vi "Get RT by Name.vi"(8 "error in":errorcluster, 10 "name":string, 11 "1553channel ref in":refnum<k24>) -> (0 "error out":errorcluster, 1 "remote terminal":refnum<k24>, 2 "found":bool, 3 "1553channel ref out":refnum<k24>)   [LabVIEW 2020, in "Ballard_1553_Hardware_ni.lvlib"]
uses:
  Ballard_1553_Hardware_ni.lvlib
  C:/Users/Administrator/Desktop/GIT/Ballard-MIL-STD-1553-Custom-Device/Source/System Explorer/SubVIs/Parse XML Ballard/1.2/BTIXML_SerDes.dll
  Ballard-MIL-STD-1553-Custom-Device/Source/System Explorer/SubVIs/Parse XML Ballard/1.2/BTIXML_SerDes.dll
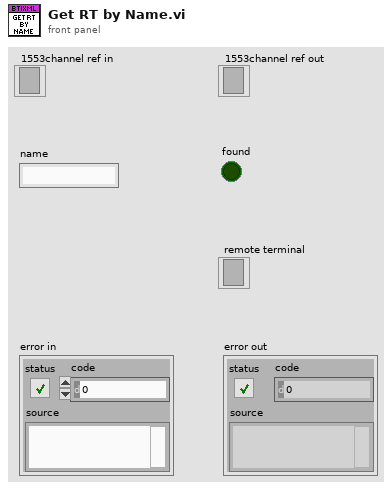
[diagram p1: front panel]
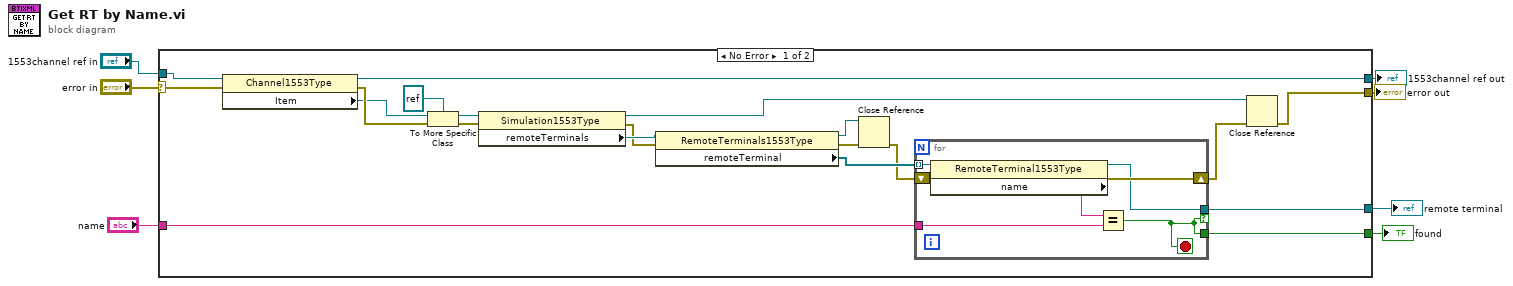
[diagram p0: block diagram]
diagram:
  n1 = case shown="No Error" "error in" {
    selector: "error in" -> [w18 w35]
    tunnel: [w19 w35] -> w7
    tunnel: [w27 w36] -> w6
    tunnel: "1553channel ref in" -> [w26 w36]
    tunnel: "name" -> [w11 _]
    tunnel: [w10 _] -> w2
    tunnel: [w8 _] -> w1
    frame No Error {
      n2 = property class="Channel1553Type"(reference=w26, error in=w18) -> (reference out=w27:refnum<k24>, error out=w25:errorcluster, "Item"=w24:refnum<k24>)
      n3 = To More Specific Class(target class=refnum<k24> refnum, reference=w24, error in=w25) -> (specific class reference=w22:refnum<k24>, error out=w21:errorcluster)
      n4 = property class="Simulation1553Type"(reference=w22, error in=w21) -> (reference out=w20:refnum<k24>, error out=w16:errorcluster, "remoteTerminals"=w17:refnum<k24>)
      n5 = property class="RemoteTerminals1553Type"(reference=w17, error in=w16) -> (reference out=w13:refnum<k24>, error out=w14:errorcluster, "remoteTerminal"=w15:refnum<k24>[])
      n6 = Close Reference(reference=w13, error in (no error)=w14) -> (error out=w12:errorcluster)
      n7 = for {
        shift-right: [w30] -> w9
        shift-left: w12 -> [w33]
        tunnel: w11 -> [w31]
        tunnel: w15 -> [w34] mode=indexing
        tunnel: [w29] -> w8 if=w28
        tunnel: [w28] -> w10
        stop <- w28 stop-if-true
        n8 = property class="RemoteTerminal1553Type"(reference=w34, error in=w33) -> (reference out=w29:refnum<k24>, error out=w30:errorcluster, "name"=w32:string)
        n9 = Equal?(x=w32, y=w31) -> (x = y?=w28:bool)
      }
      n10 = Close Reference(reference=w20, error in (no error)=w9) -> (error out=w19:errorcluster)
    }
    frame Error {
    }
  }
  "error out" <- w7
  "1553channel ref out" <- w6
  "remote terminal" <- w1
  "found" <- w2
